vi "Control Freq Test.vi"() -> ()   [LabVIEW 2021]
uses:
  <vilib>/Platform/TimedLoop/XDataNode/timing_clust.ctl
  <vilib>/Platform/TimedLoop/XDataNode/nitl_modes.ctl
  <vilib>/Platform/TimedLoop/XDataNode/wakeup.ctl
  <vilib>/DAQmx/miscellaneous.llb/DAQmx Fill In Error Info.vi
  <vilib>/platform/TimedLoop/XDataNode/XDataNode.xnode
  <vilib>/DAQmx/write.llb/DAQmx Write (Analog DBL 1Chan 1Samp).vi
  <vilib>/DAQmx/create/channels.llb/DAQmx Create Channel (AO-Voltage-Basic).vi
  <vilib>/Platform/TimedLoop/XDataNode/XDNodeRunTimeDep.lvlib
panel:
  in  "Trajectory Settings":T1={"Total Time"=10.0, "Total Length"=500.0, "Control Freq"=250.0}
  in  "stop":bool
  out "Real Time (ms)":u32
  out "Control Time (ms)":i32
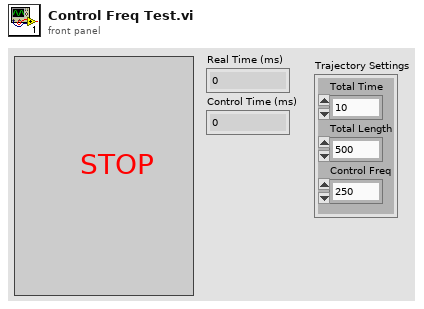
[diagram p1: front panel]
types:
  T1 = cluster{"Total Time":dbl, "Total Length":dbl, "Control Freq":dbl}
  T2 = typedef "XDNodeRunTimeDep.lvlib/timing_clust.ctl" = cluster{"Expected End [f-1]":u64, "Actual End [f-1]":u64, "Finished Late? [f-1]":bool, "Expected End [i-1]":u64, "Actual End [i-1]":u64, "Finished Late? [i-1]":bool, "Expected Start [i]":u64, "Actual Start [i]":u64, "Expected Start [f]":u64, "Actual Start [f]":u64, "Source Name":string, "Structure Name":string, "Period":i64, "Deadline":i64, "Offset":i64, "Start":i64, "Priority":i32, "Timeout":i32, "Mode":T3, "Wakeup Reason":T4, "Error":errorcluster, "Source Type":string, "Secondary Source Type":string, "Global End Time":u64, "Global Start Time":u64, "Frame Duration":u64, "Iteration Duration":u64, "Assigned CPU":i32, "I/O Scan Engine Mode":u32}
  T3 = typedef "XDNodeRunTimeDep.lvlib/nitl_modes.ctl" = enum32{"No Change", "Process missed periods, maintain original phase", "Discard missed periods, maintain original phase", "Process missed periods, ignore original phase", "Discard missed periods, ignore original phase"}
  T4 = typedef "XDNodeRunTimeDep.lvlib/wakeup.ctl" = enum32{"Normal", "Aborted", "Asynchronous wakeup", "Timing source error", "Timed loop error", "Timeout"}
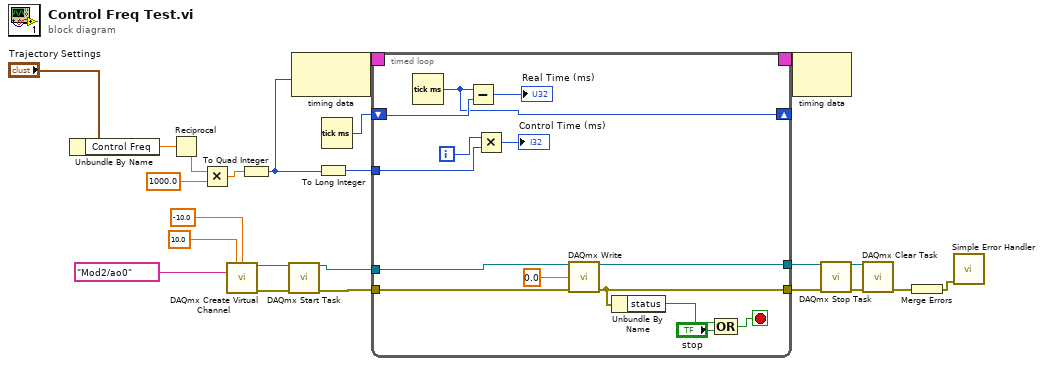
[diagram p0: block diagram]
diagram:
  n1 = Unbundle By Name("Trajectory Settings") -> ("Control Freq"=w5:dbl)
  n2 = Reciprocal(x=w5) -> (1/x=w4:dbl)
  n3 = Multiply(x=w4, y=1000.0) -> (x*y=w3:dbl)
  n4 = call-poly <vilib>:"DAQmx Create Virtual Channel.vi"("maximum value"=10.0 ("AO max"), "minimum value"=-10.0 ("AO min"), "physical channels"=tag "Mod2/ao0" ("Physical Channel(s)")) -> ("task out"=w15:refnum<k21>, "error out"=w14:errorcluster)  [unwired: 11 in]
  n5 = To Quad Integer(1:w3) -> (0:w2:i64)
  n6 = call <vilib>:"DAQmx Start Task.vi"("task/channels in"=w15, "error in"=w14) -> ("task out"=w19:refnum<k21>, "error out"=w18:errorcluster)  [unwired: 12 in]
  n7 = node-c288(w2) -> (w23:T2)
  n8 = To Long Integer(number=w2) -> (32bit integer=w1:i32)
  n9 = Tick Count (ms)() -> (millisecond timer value=w8:u32)
  n10 = timed-loop {
    tunnel: [w37] -> w21
    tunnel: [w36] -> w20
    tunnel: w19 -> [w31]
    tunnel: w18 -> [w35]
    timing: w23 -> [_]
    timing-out: [_] -> w22
    tunnel: w1 -> [w28]
    shift-right: [w25] -> _
    shift-left: w8 -> [w27]
    i -> [w30]
    stop <- w33 stop-if-true
    n11 = Tick Count (ms)() -> (millisecond timer value=w25:u32)
    n12 = Subtract(x=w25, y=w27) -> (x-y=→"Real Time (ms)":u32)
    n13 = Multiply(x=w30, y=w28) -> (x*y=→"Control Time (ms)":i32)
    n14 = call-poly <vilib>:"DAQmx Write.vi"("task/channels in"=w31, "data"=0.0, "error in"=w35) -> ("task out"=w37:refnum<k21>, "error out"=w36:errorcluster)  [unwired: 10 in, 1 out]
    n15 = Unbundle By Name(w36) -> ("status"=w34:bool)
    n16 = Compound Arithmetic op=OR(w34, "stop") -> (w33:bool)
  }
  n17 = node-c288(w22) -> ()  [unwired: 1 out]
  n18 = call <vilib>:"DAQmx Stop Task.vi"("task/channels in"=w21, "error in"=w20) -> ("task out"=w12:refnum<k21>, "error out"=w11:errorcluster)  [unwired: 12 in]
  n19 = call <vilib>:"DAQmx Clear Task.vi"("task in"=w12, "error in"=w11) -> ("error out"=w9:errorcluster)  [unwired: 13 in]
  n20 = Merge Errors(w9) -> (w10:errorcluster)
  n21 = call <vilib>:"Simple Error Handler.vi"("error in (no error)"=w10) -> ()  [unwired: 4 in, 5 out]
